vi "Filter Existing VIs.vi"(0 "Dependency Path":path[](array[path]), 11 "error in (no error)":errorcluster) -> (4 "Valid Dep Path":path[](array[path]), 15 "error out":errorcluster)   [LabVIEW 2021, in "Converter.lvlib"]
uses:
  Converter.lvlib
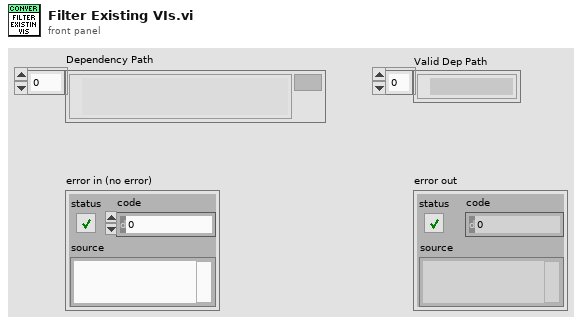
[diagram p1: front panel]
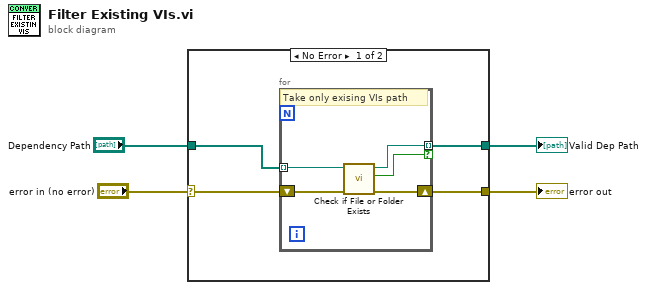
[diagram p0: block diagram]
diagram:
  n1 = case shown="No Error" "error in (no error)" {
    selector: "error in (no error)" -> [w8 w14]
    tunnel: [w7 w14] -> w3
    tunnel: "Dependency Path" -> [w6 w15]
    tunnel: [w5 w15] -> w1
    frame No Error {
      n2 = for {
        shift-right: [w12] -> w7
        shift-left: w8 -> [w13]
        tunnel: w6 -> [w11] mode=indexing
        tunnel: [w10] -> w5 mode=indexing if=w9
        # "Take only exising VIs path"
        n3 = call <vilib>:"Check if File or Folder Exists.vi"("error in (no error)"=w13, "path"=w11) -> ("error out"=w12:errorcluster, "file or folder exists?"=w9:bool, "dup path"=w10:path)  [unwired: 7 in]
      }
    }
    frame Error {
    }
  }
  "error out" <- w3
  "Valid Dep Path" <- w1
